vi "ma_sml_FFT Size and RBW (ND Zoom).vi"(0 "window":u16(ring) items=["Rectangle"=0, "Hanning"=1, "Hamming"=2, "Blackman-Harris"=3, "Exact Blackman"=4, "Blackman"=5, "Flat Top"=6, "4 Term B-Harris "=7, "7 Term B-Harris"=8, "Low Sidelobe"=9, "Blackman Nuttall"=11, "Triangle"=30, "Bartlett-Hanning"=31, "Bohman"=32, "Parzen"=33, "Welch"=34, "Kaiser"=60, "Dolph-Chebyshev"=61, "Gaussian"=62], 1 "RBW definition":enum16{"3dB", "6dB", "ENBW", "bin width"}(ring), 5 "RBW":dbl format="%.2f", 7 "zoom":dbl format="%.7f", 9 "spectral lines":i32=-1, 11 "fs":dbl format="%.2f", 12 "input signal type":enum16{"real", "complex modulated"}(ring)) -> (2 "RBW actual":dbl format="%.2f", 3 "span":dbl format="%.2f", 4 "acq. size":i32=-1, 6 "zoom factor":i32, 8 "trimming factor":dbl format="%.7f", 10 "spectral lines actual":i32=-1, 15 "FFT Size":i32=-1)   [LabVIEW 2020, in "NI_MAPro.lvlib"]
uses:
  NI_MAPro.lvlib
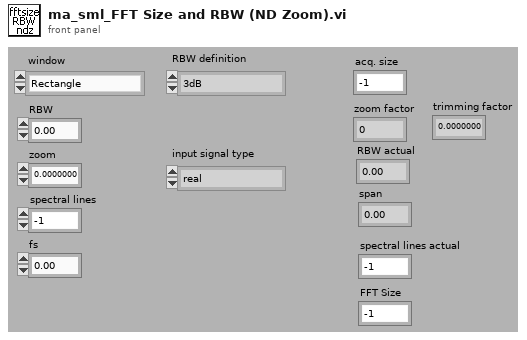
[diagram p1: front panel]
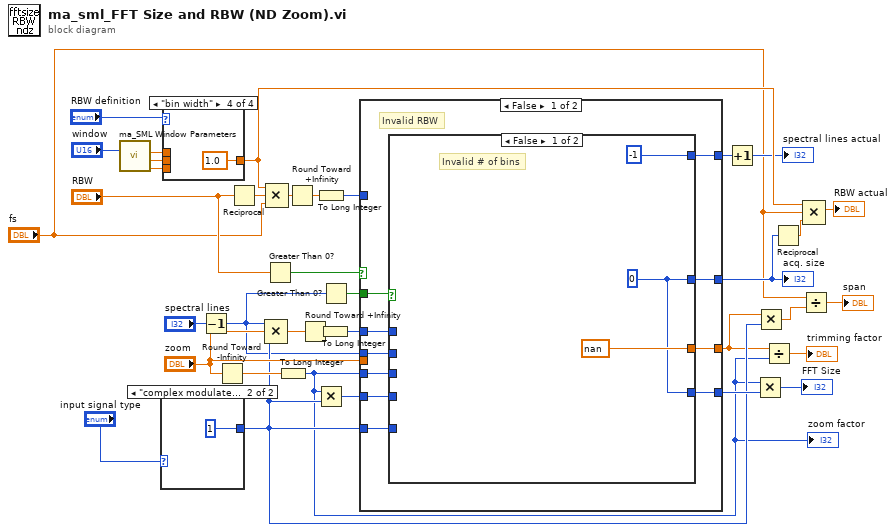
[diagram p0: block diagram]
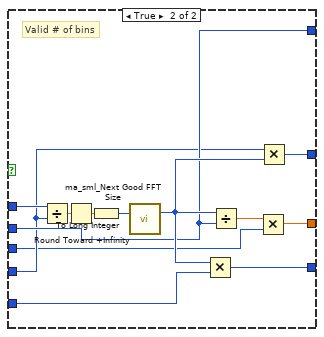
[diagram p5: hidden frame]
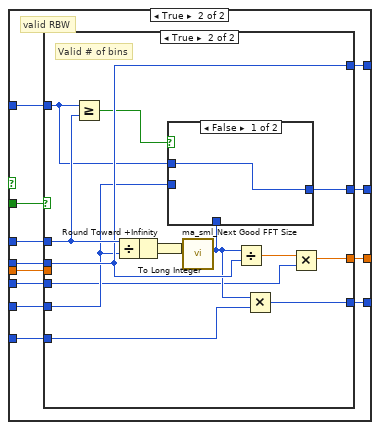
[diagram p6: hidden frame]
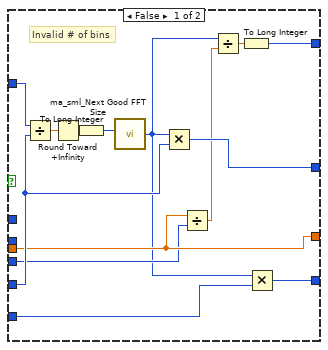
[diagram p7: hidden frame]
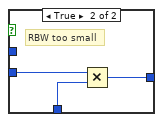
[diagram p8: hidden frame]
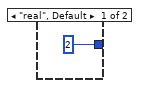
[diagram p9: hidden frame]
diagram:
  n1 = call "ma_SML Window Parameters.vi"("window"="window") -> ("ENBW"=w19:dbl, "3dB BW"=w18:dbl, "6dB BW"=w17:dbl)  [unwired: 1 out]
  n2 = case shown="\"complex modulated\"" "input signal type" {
    tunnel: [2 1] -> w26
    frame "real", Default {
    }
    frame "complex modulated" {
    }
  }
  n3 = case shown="\"bin width\"" "RBW definition" {
    tunnel: w19 -> [_ _ w41 _]
    tunnel: w18 -> [w39 _ _ _]
    tunnel: w17 -> [_ w40 _ _]
    tunnel: [w39 w40 w41 1.0 ("ENBW")] -> w15
    frame "3dB", Default {
    }
    frame "6dB" {
    }
    frame "ENBW" {
    }
    frame "bin width" {
    }
  }
  n4 = Decrement(x="spectral lines") -> (x-1=w4:i32)
  n5 = Round Toward -Infinity(1:"zoom") -> (0:w31:dbl)
  n6 = Reciprocal(x="RBW") -> (1/x=w36:dbl)
  n7 = Greater Than 0?(x="RBW") -> (x > 0?=w33:bool)
  n8 = Compound Arithmetic op=MULTIPLY(w4, "zoom", w26) -> (w10:dbl)
  n9 = Compound Arithmetic op=MULTIPLY(w15, w36, "fs") -> (w9:dbl)
  n10 = To Long Integer(number=w31) -> (32bit integer=w11:i32)
  "zoom factor" <- w11
  n11 = Round Toward +Infinity(x=w9) -> (ceil(x): smallest int >= x=w6:dbl)
  n12 = Round Toward +Infinity(x=w10) -> (ceil(x): smallest int >= x=w8:dbl)
  n13 = To Long Integer(number=w6) -> (32bit integer=w5:i32)
  n14 = Multiply(x=w11, y=w26) -> (x*y=w28:i32)
  n15 = To Long Integer(number=w8) -> (32bit integer=w7:i32)
  n16 = Greater Than 0?(x=w4) -> (x > 0?=w32:bool)
  n17 = case shown="False" w33 {
    tunnel: w5 -> [_ w79]
    tunnel: w32 -> [w52 w80]
    tunnel: w7 -> [w47 w78]
    tunnel: w28 -> [w45 w77]
    tunnel: w4 -> [w46 w76]
    tunnel: [w49 w75] -> w13
    tunnel: [w50 w74] -> w22
    tunnel: w26 -> [w44 w73]
    tunnel: [w48 w72] -> w29
    tunnel: [w51 w71] -> w3
    tunnel: "zoom" -> [_ w70]
    tunnel: w11 -> [w43 w69]
    frame False {
      # "Invalid RBW"
      n18 = case shown="False" w52 {
        tunnel: [-1 w61] -> w51
        tunnel: [w53 w63] -> w50
        tunnel: [nan w59] -> w49
        tunnel: [w53 w64] -> w48
        tunnel: w47 -> [_ w66]
        tunnel: w46 -> [_ w61]
        tunnel: w45 -> [_ w60]
        tunnel: w44 -> [_ w65]
        tunnel: w43 -> [_ w58]
        frame False {
          w53 = 0
          # "Invalid # of bins"
        }
        frame True {
          # "Valid # of bins"
          n19 = Divide(x=w66, y=w60) -> (x/y=w67:dbl)
          n20 = Round Toward +Infinity(x=w67) -> (ceil(x): smallest int >= x=w57:dbl)
          n21 = To Long Integer(number=w57) -> (32bit integer=w56:i32)
          n22 = call "ma_sml_Next Good FFT Size.vi"("FFT Size"=w56) -> ("least bigger good size"=w62:i32)
          n23 = Multiply(x=w62, y=w65) -> (x*y=w64:i32)
          n24 = Divide(x=w62, y=w61) -> (x/y=w68:dbl)
          n25 = Multiply(x=w68, y=w58) -> (x*y=w59:dbl)
          n26 = Multiply(x=w60, y=w62) -> (x*y=w63:i32)
        }
      }
    }
    frame True {
      # "valid RBW"
      n27 = case shown="True" w80 {
        tunnel: w79 -> [w94 w101]
        tunnel: w78 -> [_ w109]
        tunnel: w77 -> [w92 w100]
        tunnel: w76 -> [_ w105]
        tunnel: [w88 w98] -> w75
        tunnel: [w91 w108] -> w74
        tunnel: w73 -> [w83 w107]
        tunnel: [w85 w106] -> w72
        tunnel: [w89 w105] -> w71
        tunnel: w70 -> [w88 _]
        tunnel: w69 -> [w87 w97]
        frame False {
          # "Invalid # of bins"
          n28 = Divide(x=w94, y=w92) -> (x/y=w93:dbl)
          n29 = Round Toward +Infinity(x=w93) -> (ceil(x): smallest int >= x=w82:dbl)
          n30 = To Long Integer(number=w82) -> (32bit integer=w81:i32)
          n31 = call "ma_sml_Next Good FFT Size.vi"("FFT Size"=w81) -> ("least bigger good size"=w84:i32)
          n32 = Multiply(x=w84, y=w92) -> (x*y=w91:i32)
          n33 = Divide(x=w88, y=w87) -> (x/y=w86:dbl)
          n34 = Divide(x=w84, y=w86) -> (x/y=w90:dbl)
          n35 = To Long Integer(number=w90) -> (32bit integer=w89:i32)
          n36 = Multiply(x=w84, y=w83) -> (x*y=w85:i32)
        }
        frame True {
          # "Valid # of bins"
          n37 = Greater Or Equal?(x=w101, y=w109) -> (x >= y?=w102:bool)
          n38 = Divide(x=w109, y=w100) -> (x/y=w104:dbl)
          n39 = Round Toward +Infinity(x=w104) -> (ceil(x): smallest int >= x=w96:dbl)
          n40 = To Long Integer(number=w96) -> (32bit integer=w95:i32)
          n41 = call "ma_sml_Next Good FFT Size.vi"("FFT Size"=w95) -> ("least bigger good size"=w103:i32)
          n42 = case shown="False" w102 {
            tunnel: w100 -> [_ w113]
            tunnel: [w110 w112] -> w108
            tunnel: w103 -> [_ w111]
            tunnel: w101 -> [w110 _]
            frame False {
            }
            frame True {
              # "RBW too small"
              n43 = Multiply(x=w113, y=w111) -> (x*y=w112:i32)
            }
          }
          n44 = Divide(x=w103, y=w105) -> (x/y=w99:dbl)
          n45 = Multiply(x=w103, y=w107) -> (x*y=w106:i32)
          n46 = Multiply(x=w99, y=w97) -> (x*y=w98:dbl)
        }
      }
    }
  }
  "acq. size" <- w22
  n47 = Increment(x=w3) -> (x+1=→"spectral lines actual":i32)
  n48 = Multiply(x=w11, y=w29) -> (x*y=→"FFT Size":i32)
  n49 = Multiply(x=w13, y=w26) -> (x*y=w14:dbl)
  n50 = Divide(x=w13, y=w11) -> (x/y=→"trimming factor":dbl)
  n51 = Reciprocal(x=w22) -> (1/x=w16:dbl)
  n52 = Divide(x="fs", y=w14) -> (x/y=→"span":dbl)
  n53 = Compound Arithmetic op=MULTIPLY(w15, "fs", w16) -> (→"RBW actual":dbl)
